vi "rad_RT Image Compare Dialog.vi"(5 "App Images Repository":path=path "c:/checksums.bin", 6 "Begin Automatically? (F)":bool, 7 "Temp Folder":path=path "C:/AppImages/_temp", 8 "error in (no error)":errorcluster, 9 "Operation":T4=enum."Compare Two Local Images", 10 "Target settings":T1={"Hostname"="", "Serial number"="", "Product name"="", "Product code"=0, "System status"="", "Credential type"=enum."None/Unlocked", "User added?"=FALSE, "Primary NIC"={"MAC address"="", "IP Address Request Mode"=2, "IP address"="", "Subnet mask"="", "Gateway"="", "DNS server"=""}} {"Primary NIC"."IP Address Request Mode" items=["Static"=1, "DHCP/Link-Local"=2, "Link-Local Only"=4, "DHCP Only"=8]}, 11 "Original Image Path":path) -> (0 "error out":errorcluster)   [LabVIEW 2020]
uses:
  TypeDefs/rad_Comparison Modes.ctl
  Targets/TypeDefs/rad_Target Information.ctl
  Targets/TypeDefs/rad_Target Network Settings.ctl
  Util/FP Control/FP Control Functions.ctl
  <vilib>/Utility/miscctls.llb/LVRowAndColumnUnsignedTypeDef.ctl
panel:
  in  "Compare Images":bool
  out "Results Table":i32(listbox)
  in  "Exit Notifier":bool
  in  "Ignore Automatically Updated Files":bool=TRUE
  in  "Comparison Image Path":path=path "c:/checksums.bin"
  in  "State Variables":T3
  in  "RT Target IP":string caption="RT Target - IP Address or Name"
  in  "Close":bool
  in  "Compare Files":bool
  # "Red software indicates different components"
  # "Blue software indicates different versions"
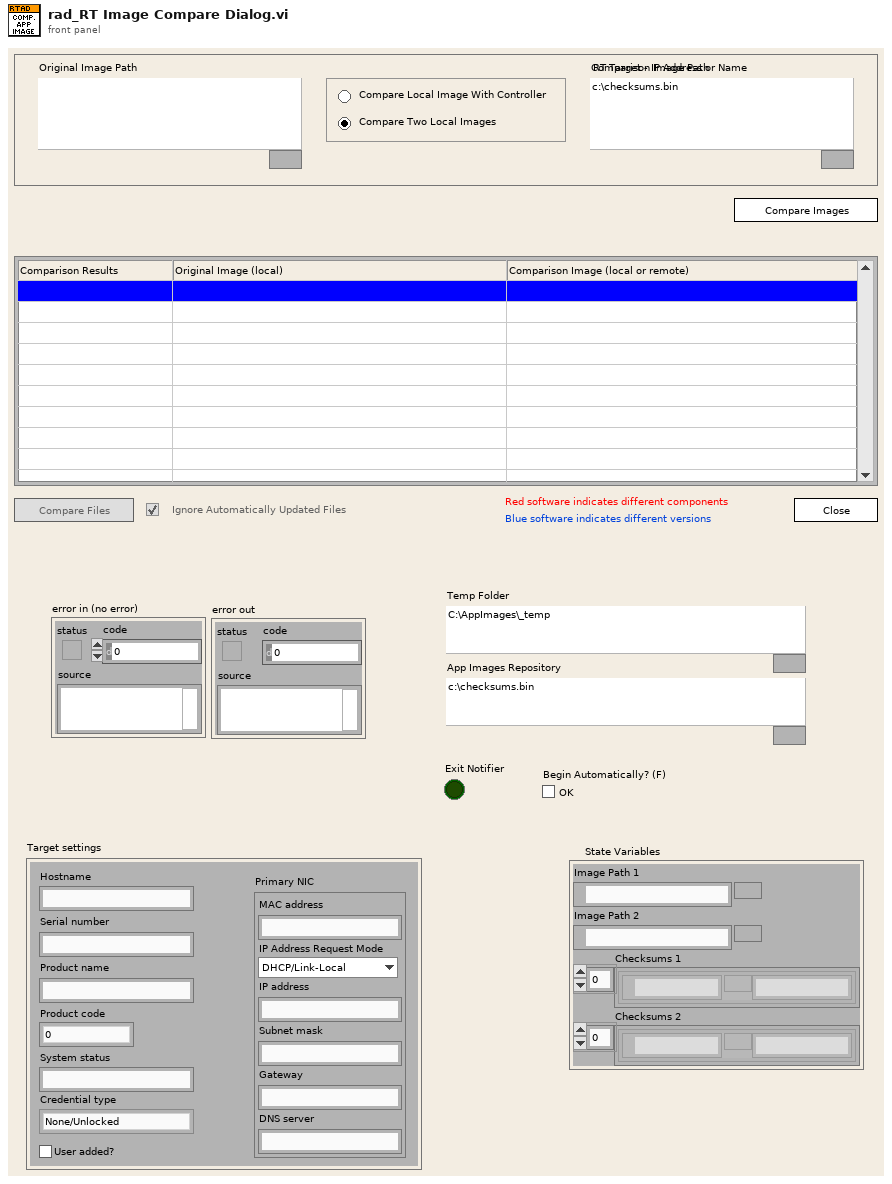
[diagram p1: front panel]
types:
  T1 = typedef "rad_Target Information.ctl" = cluster{"Hostname":string, "Serial number":string, "Product name":string, "Product code":i32, "System status":string, "Credential type":enum16{"None/Unlocked", "FTP Password", "NIAuth Credentials"}, "User added?":bool, "Primary NIC":T2}
  T2 = typedef "rad_Target Network Settings.ctl" = cluster{"MAC address":string, "IP Address Request Mode":i32, "IP address":string, "Subnet mask":string, "Gateway":string, "DNS server":string}
  T3 = cluster{"Image Path 1":path, "Image Path 2":path, "Checksums 1":cluster{path, string}[], "Checksums 2":cluster{path, string}[]}
  T4 = typedef "rad_Comparison Modes.ctl" = enum32{"Compare Local Image With Controller", "Compare Two Local Images"}
  T5 = typedef "LVRowAndColumnUnsignedTypeDef.ctl" = cluster{"Row":u32, "Column":u32}
  T6 = typedef "FP Control Functions.ctl" = enum16{"Open", "Close", "Bring To Front", "Center"}
  T7 = enum8{"Enabled", "Disabled", "Disabled and Grayed Out"}
  T8 = typedef "rad_Application Image Properties.ctl" = cluster{"Name":string, "Version":string, "Time":timestamp, "Description":string, "Key":string, "Chassis":string, "FPGA Properties":T9, "Model":string, "Retrieve":string[], "Deploy":string[], "Installed Software":string[]}
  T9 = typedef "rad_FPGA Properties.ctl" = T10[]
  T10 = typedef "rad_FPGA Flash Properties.ctl" = cluster{"Resource Name":string, "Path":path}
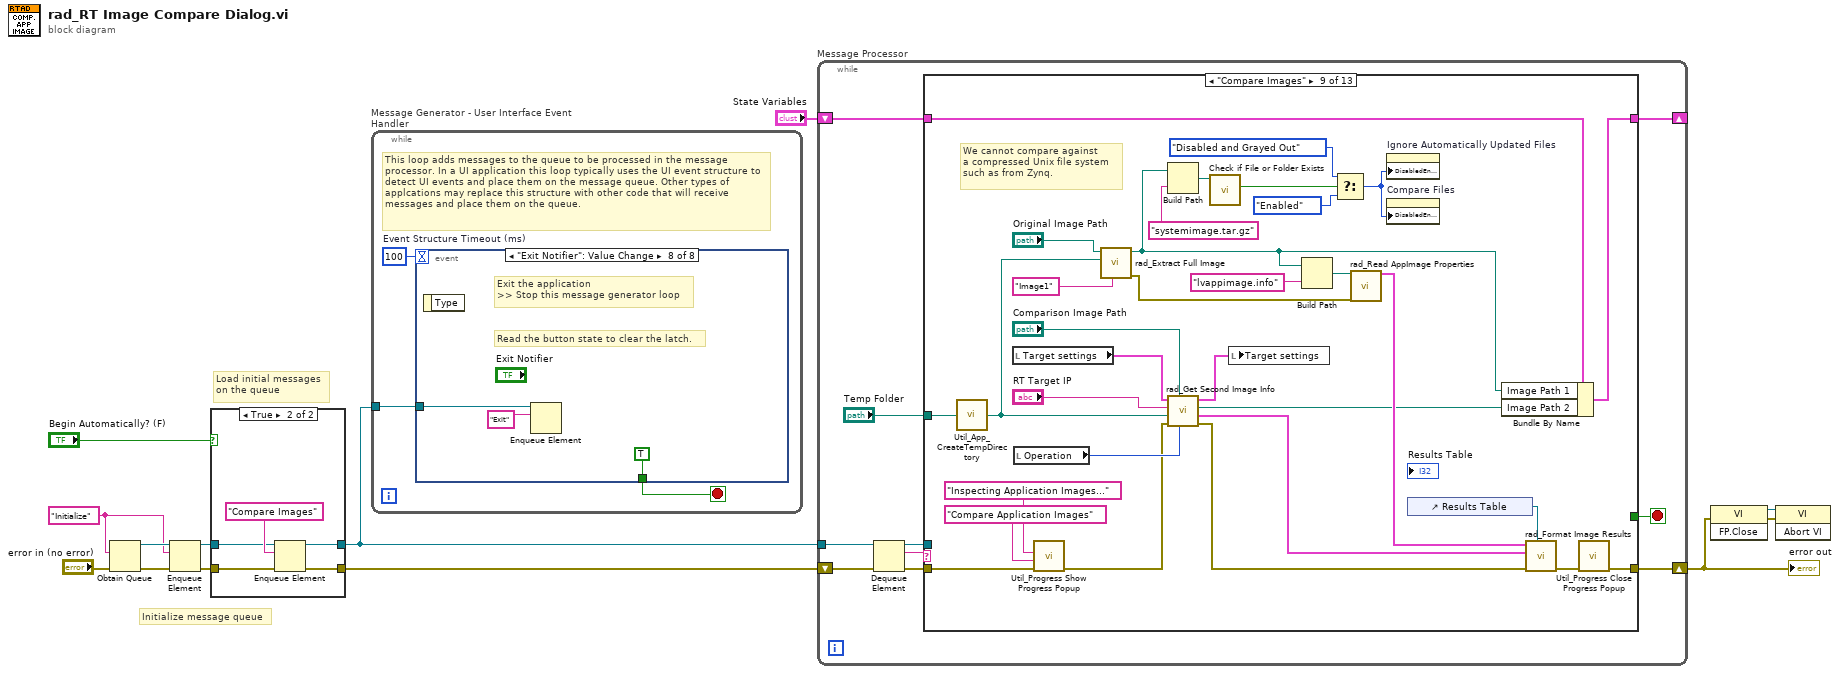
[diagram p0: block diagram]
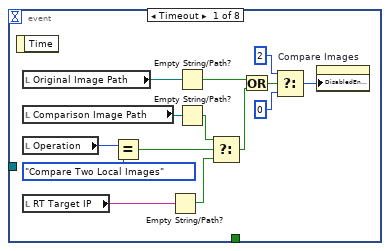
[diagram p3: hidden frame]
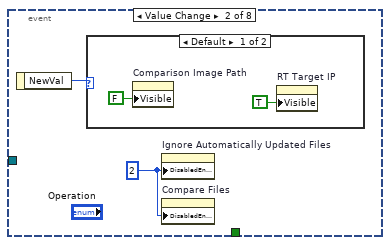
[diagram p4: hidden frame]
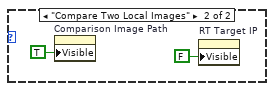
[diagram p5: hidden frame]
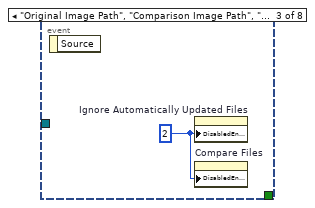
[diagram p6: hidden frame]
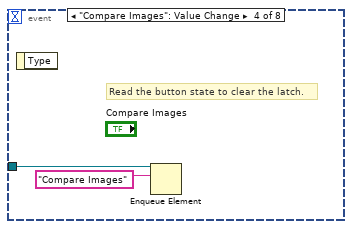
[diagram p7: hidden frame]
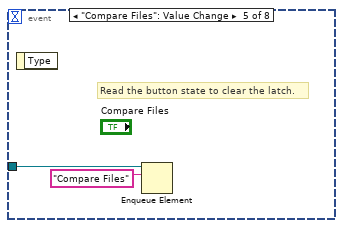
[diagram p8: hidden frame]
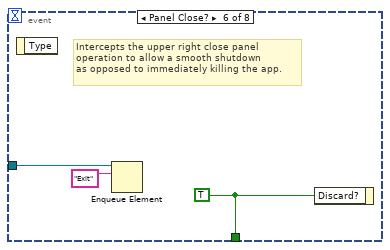
[diagram p9: hidden frame]
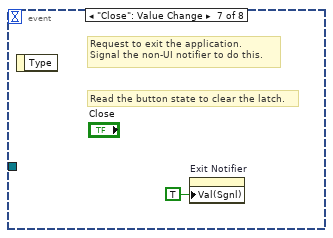
[diagram p10: hidden frame]
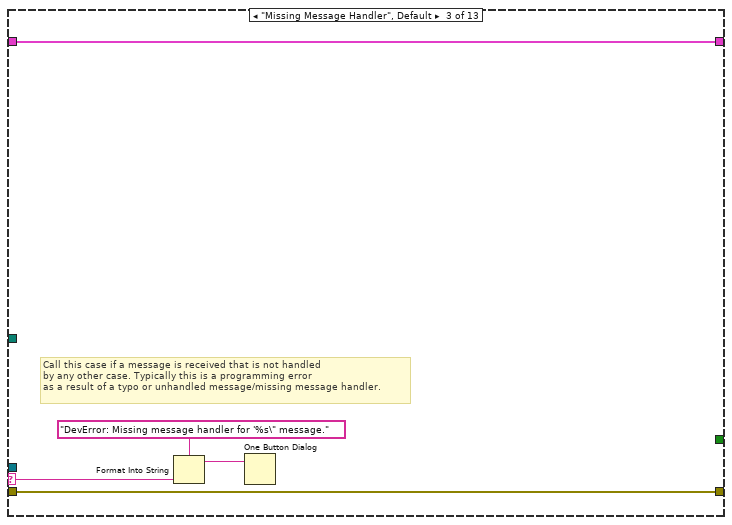
[diagram p13: hidden frame]
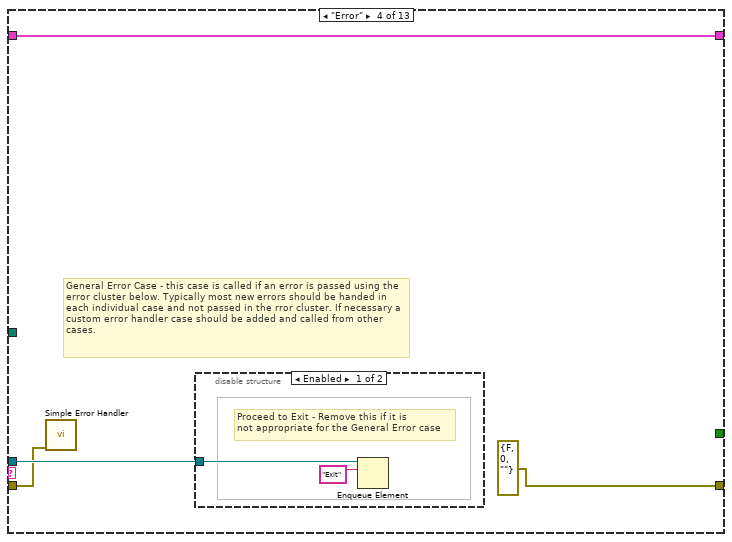
[diagram p14: hidden frame]
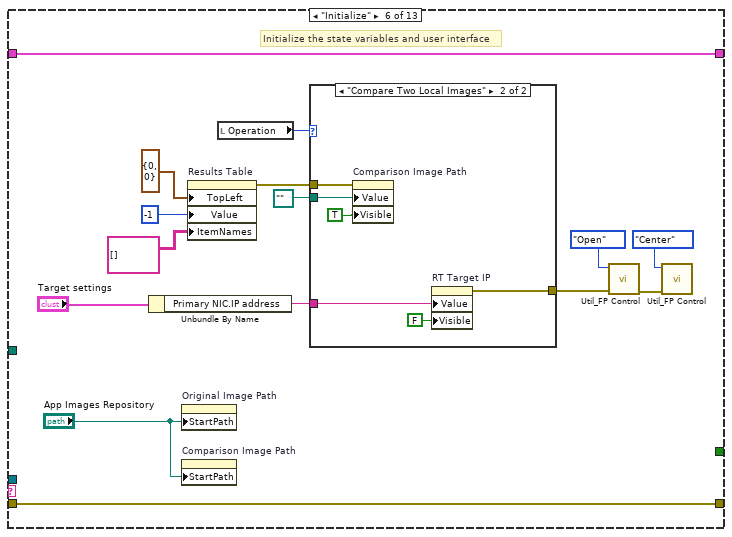
[diagram p17: hidden frame]
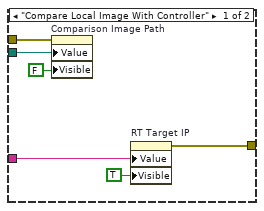
[diagram p18: hidden frame]
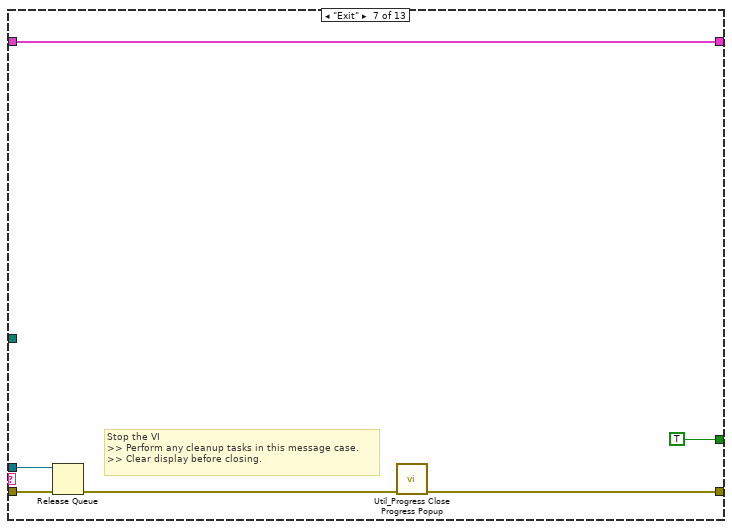
[diagram p19: hidden frame]
diagram:
  w5 = "Initialize"
  # "Initialize message queue"
  # "Load initial messages\non the queue"
  n1 = Obtain Queue(element data type=w5, error in (no error)="error in (no error)") -> (queue out=w7:refnum<queue>, error out=w6:errorcluster)  [unwired: 3 in, 1 out]
  n2 = Enqueue Element(queue=w7, element=w5, error in (no error)=w6) -> (queue out=w4:refnum<queue>, error out=w3:errorcluster)  [unwired: 1 in, 1 out]
  n3 = case shown="True" "Begin Automatically? (F)" {
    tunnel: w4 -> [w14 w19]
    tunnel: w3 -> [w15 w16]
    tunnel: [w15 w17] -> w2
    tunnel: [w14 w18] -> w1
    frame False {
    }
    frame True {
      n4 = Enqueue Element(queue=w19, element="Compare Images", error in (no error)=w16) -> (queue out=w18:refnum<queue>, error out=w17:errorcluster)  [unwired: 1 in, 1 out]
    }
  }
  n5 = while "Message Generator - User Interface Event Handler" {
    tunnel: w1 -> [w21]
    stop <- w22 stop-if-true
    w23 = 100  # Event Structure Timeout (ms)
    # "This loop adds messages to the queue to be processed in the message processor. In a UI application this loop typically uses the UI event structure to detect UI events and place them on the message queue. Other types of applcations may replace this structure with other code that will receive messages and place them on the queue."
    n6 = event shown="[7] \"Exit Notifier\": Value Change" {
      selector: _ -> [_ _ _ _ _ _ _ _]
      dyn-events: _ -> [_ _ _ _ _ _ _ _]
      timeout: w23 -> [_ _ _ _ _ _ _ _]
      tunnel: [_ _ _ _ _ w51 _ TRUE ("Discard?")] -> w22
      tunnel: w21 -> [_ _ _ w45 w48 w49 _ w53]
      event Timeout {
        n7 = event-data() -> ()  [unwired: 2 out]
        n8 = local read "Original Image Path"() -> (w27:path)
        n9 = local read "Comparison Image Path"() -> (w24:path)
        n10 = local read "Operation"() -> (w37:T4)
        n11 = local read "RT Target IP"() -> (w28:string)
        n12 = Equal?(x=w37, y=rad_Comparison_Modes."Compare Two Local Images") -> (x = y?=w35:bool)
        n13 = Empty String/Path?(string/path=w28) -> (empty?=w29:bool)
        n14 = Empty String/Path?(string/path=w27) -> (empty?=w26:bool)
        n15 = Empty String/Path?(string/path=w24) -> (empty?=w25:bool)
        n16 = Select(t=w25, s=w35, f=w29) -> (s? t:f=w34:bool)
        n17 = Or(x=w26, y=w34) -> (x .or. y?=w33:bool)
        n18 = Select(t=2, s=w33, f=0) -> (s? t:f=w30:i32)
        n19 = property on="Compare Images" class="Bool"("DisabledEnum"=w30) -> ()  [unwired: 2 in, 2 out]
      }
      event Value Change {
        w38 = 2
        n20 = event-data() -> ("NewVal"=w39:T4)  [unwired: 1 out]
        n21 = case shown="Default" w39 {
          frame Default {
            n22 = property on="Comparison Image Path" class="Path"("Visible"=FALSE) -> ()  [unwired: 2 in, 2 out]
            n23 = property on="RT Target IP" class="Str"("Visible"=TRUE) -> ()  [unwired: 2 in, 2 out]
          }
          frame "Compare Two Local Images" {
            n24 = property on="Comparison Image Path" class="Path"("Visible"=TRUE) -> ()  [unwired: 2 in, 2 out]
            n25 = property on="RT Target IP" class="Str"("Visible"=FALSE) -> ()  [unwired: 2 in, 2 out]
          }
        }
        n26 = property on="Ignore Automatically Updated Files" class="Bool (strict)"("DisabledEnum"=w38) -> ()  [unwired: 2 in, 2 out]
        n27 = property on="Compare Files" class="Bool"("DisabledEnum"=w38) -> ()  [unwired: 2 in, 2 out]
      }
      event "Original Image Path", "Comparison Image Path", "RT Target IP": Value Change {
        w44 = 2
        n28 = event-data() -> ()  [unwired: 2 out]
        n29 = property on="Ignore Automatically Updated Files" class="Bool (strict)"("DisabledEnum"=w44) -> ()  [unwired: 2 in, 2 out]
        n30 = property on="Compare Files" class="Bool"("DisabledEnum"=w44) -> ()  [unwired: 2 in, 2 out]
      }
      event "Compare Images": Value Change {
        # "Read the button state to clear the latch."
        n31 = event-data() -> ()  [unwired: 2 out]
        n32 = Enqueue Element(queue=w45, element="Compare Images") -> ()  [unwired: 2 in, 3 out]
      }
      event "Compare Files": Value Change {
        # "Read the button state to clear the latch."
        n33 = event-data() -> ()  [unwired: 2 out]
        n34 = Enqueue Element(queue=w48, element="Compare Files") -> ()  [unwired: 2 in, 3 out]
      }
      event Panel Close? {
        w51 = TRUE ("Discard?")
        # "Intercepts the upper right close panel\noperation to allow a smooth shutdown\nas opposed to immediately killing the app."
        n35 = event-data() -> ()  [unwired: 2 out]
        n36 = Enqueue Element(queue=w49, element="Exit") -> ()  [unwired: 2 in, 3 out]
        n37 = event-data("Discard?"=w51) -> ()  [unwired: 1 in, 1 out]
      }
      event "Close": Value Change {
        # "Read the button state to clear the latch."
        # "Request to exit the application.\nSignal the non-UI notifier to do this."
        n38 = event-data() -> ()  [unwired: 2 out]
        n39 = property on="Exit Notifier" class="Bool (strict)"("Val(Sgnl)"=TRUE ("Value (Signaling)")) -> ()  [unwired: 2 in, 2 out]
      }
      event "Exit Notifier": Value Change {
        # "Read the button state to clear the latch."
        # "Exit the application\n>> Stop this message generator loop"
        n40 = event-data() -> ()  [unwired: 2 out]
        n41 = Enqueue Element(queue=w53, element="Exit") -> ()  [unwired: 2 in, 3 out]
      }
    }
  }
  n42 = while "Message Processor" {
    shift-left: w2 -> [w60]
    shift-right: [w63] -> w8
    tunnel: w1 -> [w61]
    shift-left: "State Variables" -> [w65]
    shift-right: [w64] -> _
    stop <- w56 stop-if-true
    n43 = Dequeue Element(queue=w61, error in (no error)=w60) -> (queue out=w62:refnum<queue>, element=w58:string, error out=w59:errorcluster)  [unwired: 1 in, 1 out]
    n44 = case shown="\"Compare Images\"" w58 {
      selector: w58 -> [_ _ w72 _ _ _ _ _ _ _ _ _ _]
      tunnel: [w67 w69 w74 w78 w82 w97 w115 w117 w148 w150 w192 w208 w216] -> w64
      tunnel: w65 -> [w67 w69 w74 w78 w82 w97 w115 w117 w149 w150 w193 w208 w216]
      tunnel: w62 -> [_ _ _ w76 _ _ w113 _ _ w153 w191 w207 _]
      tunnel: w59 -> [w66 w68 w73 w75 w81 w96 w114 w116 w125 w156 w181 w194 w217]
      tunnel: [w66 w68 w73 errorcluster {"status"=FALSE, "code"=0, "source"=""} ("error out") w81 w96 w111 w116 w126 w155 w183 w199 w213] -> w63
      tunnel: "Temp Folder" -> [_ _ _ _ _ _ _ _ w145 _ _ _ w219]
      tunnel: [_ _ _ _ _ _ TRUE _ _ _ _ _ _] -> w56
      frame "---------- Framework Operations ----------" {
        # "Dummy case to add a seperator in the Case Structure menu"
      }
      frame "", "Idle" {
        # "Idle Case - this case is called after a Timeout on the Get Next Message from Queue VI, if no new messages are present on the queue. This case can be used for housekeeping tasks such as updating the UI."
      }
      frame "Missing Message Handler", Default {
        # "Call this case if a message is received that is not handled \nby any other case. Typically this is a programming error\nas a result of a typo or unhandled message/missing message handler."
        n45 = Format Into String(format string="DevError: Missing message handler for '%s\" message." ("message"), w72) -> (resulting string=w70:string)  [unwired: 2 in, 1 out]
        n46 = One Button Dialog(message=w70) -> ()  [unwired: 2 out]
      }
      frame "Error" {
        # "General Error Case - this case is called if an error is passed using the error cluster below. Typically most new errors should be handed in each individual case and not passed in the rror cluster. If necessary a custom error handler case should be added and called from other cases."
        n47 = call <vilib>:"Simple Error Handler.vi"("error in (no error)"=w75) -> ()  [unwired: 1 in, 8 out]
        n48 = disable-structure shown="Enabled" {
          disable-tunnel: w76 -> [w80 _]
          frame Enabled {
            # "Proceed to Exit - Remove this if it is\nnot appropriate for the General Error case"
            n49 = Enqueue Element(queue=w80, element="Exit") -> ()  [unwired: 2 in, 3 out]
          }
          frame Disabled {
          }
        }
      }
      frame "---------- Generic Operations ----------" {
        # "Dummy case to add a seperator in the Case Structure menu"
      }
      frame "Initialize" {
        # "Initialize the state variables and user interface"
        n50 = Unbundle By Name("Target settings") -> ("Primary NIC.IP address"=w87:string)
        n51 = property on="Original Image Path" class="Path"("StartPath"="App Images Repository") -> ()  [unwired: 2 in, 2 out]
        n52 = property on="Comparison Image Path" class="Path"("StartPath"="App Images Repository") -> ()  [unwired: 2 in, 2 out]
        n53 = property on="Results Table" class="MCListbox (strict)"("TopLeft"=T5 {"Row"=0, "Column"=0} ("Top Left Visible Cell"), "Value"=-1 ("Results Table"), "ItemNames"=string[][] [] ("Item Names")) -> (error out=w83:errorcluster)  [unwired: 2 in, 1 out]
        n54 = local read "Operation"() -> (w88:T4)
        n55 = case shown="\"Compare Two Local Images\"" w88 {
          tunnel: [w103 w109] -> w93
          tunnel: path "" ("Value (Signaling)") -> [w100 w106]
          tunnel: w87 -> [w99 w105]
          tunnel: w83 -> [w98 w104]
          frame "Compare Local Image With Controller" {
            n56 = property on="Comparison Image Path" class="Path"(error in=w98, "Value"=w100, "Visible"=FALSE) -> ()  [unwired: 1 in, 2 out]
            n57 = property on="RT Target IP" class="Str"("Value"=w99, "Visible"=TRUE) -> (error out=w103:errorcluster)  [unwired: 2 in, 1 out]
          }
          frame "Compare Two Local Images" {
            n58 = property on="Comparison Image Path" class="Path"(error in=w104, "Value"=w106, "Visible"=TRUE) -> ()  [unwired: 1 in, 2 out]
            n59 = property on="RT Target IP" class="Str"("Value"=w105, "Visible"=FALSE) -> (error out=w109:errorcluster)  [unwired: 2 in, 1 out]
          }
        }
        n60 = call "Util_FP Control.vi"("error in (no error)"=w93, "Function"=FP_Control_Functions."Open") -> ("error out"=w91:errorcluster)  [unwired: 9 out]
        n61 = call "Util_FP Control.vi"("error in (no error)"=w91, "Function"=FP_Control_Functions."Center") -> ()  [unwired: 10 out]
      }
      frame "Exit" {
        # "Stop the VI\n>> Perform any cleanup tasks in this message case.\n>> Clear display before closing."
        n62 = Release Queue(queue=w113, error in (no error)=w114) -> (error out=w112:errorcluster)  [unwired: 1 in, 2 out]
        n63 = call "Util_Progress Close Progress Popup.vi"("error in (no error)"=w112) -> ("error out"=w111:errorcluster)  [unwired: 10 in]
      }
      frame "---------- Application Operations ----------" {
        # "Dummy case to add a seperator in the Case Structure menu"
      }
      frame "Compare Images" {
        # "We cannot compare against\na compressed Unix file system\nsuch as from Zynq."
        n64 = call "Util_App_CreateTempDirectory.vi"("TempFolderPath"=w145) -> ("TempFolderPath_out"=w135:path)
        n65 = local read "Target settings"() -> (w122:T1)
        n66 = local read "Operation"() -> (w144:T4)
        n67 = call "Util_Progress Show Progress Popup.vi"("error in (no error)"=w125, "Title"="Compare Application Images", "Message"="Inspecting Application Images...") -> ("error out"=w124:errorcluster)  [unwired: 8 in]
        n68 = call "rad_Extract Full Image.vi"("Subfolder (lvappimage.contents)"="Image1" ("name or relative path"), "App Image Temp Folder"=w135, "Zipped App Image File Path"="Original Image Path") -> ("error out"=w123:errorcluster, "Unzipped App Image Folder Path"=w128:path)  [unwired: 7 in]
        n69 = Build Path(base path=w128, name or relative path="systemimage.tar.gz") -> (appended path=w131:path)
        n70 = call "rad_Get Second Image Info.vi"("Operation"=w144, "Comparison Image Path"="Comparison Image Path", "error in (no error)"=w124, "TempFolder Path"=w135, "RT Target IP"="RT Target IP", "Target settings in"=w122) -> ("error out"=w141:errorcluster, "AppImage Properties"=w120:T8, "Unzipped App Image Folder Path"=w119:path, "Target settings out"=w118:T1)  [unwired: 2 in]
        n71 = call <vilib>:"Check if File or Folder Exists.vi"("path"=w131) -> ("file or folder exists?"=w130:bool)  [unwired: 8 in, 2 out]
        n72 = local write "Target settings"(w118) -> ()
        n73 = Build Path(base path=w128, name or relative path="lvappimage.info") -> (appended path=w138:path)
        n74 = Select(t=T7."Disabled and Grayed Out" ("Disabled"), s=w130, f=T7."Enabled" ("Disabled")) -> (s? t:f=w134:T7)
        n75 = call "rad_Read AppImage Properties.vi"("AppImage Properties Path"=w138, "error in (no error)"=w123) -> ("AppImage Properties"=w137:T8)  [unwired: 12 in, 5 out]
        n76 = property on="Ignore Automatically Updated Files" class="Bool (strict)"("DisabledEnum"=w134) -> ()  [unwired: 2 in, 2 out]
        n77 = property on="Compare Files" class="Bool"("DisabledEnum"=w134) -> ()  [unwired: 2 in, 2 out]
        n78 = control-ref of="Results Table"() -> (w140:refnum<vi>)
        n79 = Bundle By Name(cluster=w149, "Image Path 1"=w128, "Image Path 2"=w119) -> (w148:T3)
        n80 = call "rad_Format Image Results.vi"("Results listbox"=w140, "error in (no error)"=w141, "AppImage 2"=w120, "AppImage 1"=w137) -> ("error out"=w127:errorcluster)  [unwired: 7 in]
        n81 = call "Util_Progress Close Progress Popup.vi"("error in (no error)"=w127) -> ("error out"=w126:errorcluster)  [unwired: 10 in]
      }
      frame "Compare Files" {
        n82 = local read "Operation"() -> (w151:T4)
        n83 = call "Util_Progress Show Progress Popup.vi"("error in (no error)"=w156, "Title"="Compare Application Images", "Message"="Inspecting File Systems...") -> ()  [unwired: 8 in, 1 out]
        n84 = case shown="\"Compare Local Image With Controller\"" w151 {
          tunnel: [w176 w178] -> w154
          tunnel: w156 -> [w177 w178]
          tunnel: [w175 _] -> w152
          tunnel: w150 -> [w174 _]
          frame "Compare Local Image With Controller" {
            # "The original image was already\nexpanded, but we still need to\nget the target's image."
            n85 = Unbundle By Name(w174) -> ("Image Path 2"=w173:path)
            n86 = local read "Target settings"() -> (w172:T1)
            n87 = call "rad_Retrieve Image Wrapper.vi"("error in (no error)"=w177, "image file path"=w173, "Target settings"=w172) -> ("error out"=w176:errorcluster, "Canceled"=w175:bool)  [unwired: 7 in]
          }
          frame "Compare Two Local Images" {
            # "Both file systems were\nalready expanded during the\nCompare Images step."
          }
        }
        n88 = case shown="No Error" w154 {
          selector: w154 -> [w161 w171]
          tunnel: [w162 w171] -> w155
          tunnel: w153 -> [w160 _]
          tunnel: w152 -> [w159 _]
          frame No Error {
            n89 = case shown="False" w159 {
              tunnel: [w165 w169] -> w162
              tunnel: w161 -> [w164 w170]
              tunnel: w160 -> [w163 w167]
              frame False {
                n90 = Enqueue Element(queue=w163, element="Create Checksums", error in (no error)=w164) -> (error out=w165:errorcluster)  [unwired: 1 in, 2 out]
              }
              frame True {
                n91 = Enqueue Element(queue=w167, element="Cleanup", error in (no error)=w170) -> (error out=w169:errorcluster)  [unwired: 1 in, 2 out]
              }
            }
          }
          frame Error {
          }
        }
      }
      frame "Create Checksums" {
        n92 = Unbundle By Name(w193) -> ("Image Path 1"=w179:path, "Image Path 2"=w180:path)
        n93 = call "rad_Calculate Checksum.vi"("error in"=w181, "Ignore tmp Files"="Ignore Automatically Updated Files", "Image Base Folder"=w179) -> ("error out"=w185:errorcluster, "Checksums"=w189:cluster{path, "MD5 message-digest":string}[])  [unwired: 6 in, 1 out]
        n94 = call "rad_Calculate Checksum.vi"("error in"=w181, "Ignore tmp Files"="Ignore Automatically Updated Files", "Image Base Folder"=w180) -> ("error out"=w186:errorcluster, "Checksums"=w188:cluster{path, "MD5 message-digest":string}[])  [unwired: 6 in, 1 out]
        n95 = Enqueue Element(queue=w191, element="Compare" ("Message Name"), error in (no error)=w181) -> (error out=w187:errorcluster)  [unwired: 1 in, 2 out]
        n96 = Bundle By Name(cluster=w193, "Checksums 1"=w189, "Checksums 2"=w188) -> (w192:T3)
        n97 = Merge Errors(w185, w186, w187) -> (w182:errorcluster)
        n98 = call "Util_Progress Close Progress Popup.vi"("error in (no error)"=w182) -> ("error out"=w183:errorcluster)  [unwired: 10 in]
      }
      frame "Compare" {
        n99 = call "Util_Progress Show Progress Popup.vi"("error in (no error)"=w194, "Title"="Compare Application Images", "Message"="Comparing Application Checksums...") -> ("error out"=w195:errorcluster)  [unwired: 8 in]
        n100 = Unbundle By Name(w208) -> ("Checksums 1"=w204:cluster{path, string}[], "Checksums 2"=w205:cluster{path, string}[])
        n101 = Enqueue Element(queue=w207, element="Cleanup" ("Message Name"), error in (no error)=w195) -> (error out=w199:errorcluster)  [unwired: 1 in, 2 out]
        n102 = call "rad_Compare Checksums.vi"("Checksums 2"=w205, "Checksums 1"=w204) -> ("Files In 2 Only"=w200:path[], "Files In 1 Only"=w201:path[], "Modified Files"=w202:path[], "Identical?"=w203:bool)  [unwired: 6 out]
        n103 = call "Util_Progress Close Progress Popup.vi"("error in (no error)"=w199) -> ("error out"=w198:errorcluster)  [unwired: 10 in]
        n104 = case shown="False" w203 {
          tunnel: w202 -> [w211 _]
          tunnel: w201 -> [w210 _]
          tunnel: w200 -> [w209 _]
          tunnel: w198 -> [_ _]
          frame False {
            n105 = call "rad_View Comparison Results.vi"("Files Found Only In New Image"=w209, "Files Found Only In Original Image"=w210, "Modified Files"=w211) -> ()  [unwired: 8 in, 1 out]
          }
          frame True {
            n106 = One Button Dialog(message="RT Image Verified Successfully.\nThe Two Images Are Identical.") -> ()  [unwired: 1 in, 1 out]
          }
        }
      }
      frame "Cleanup" {
        n107 = Delete(path (use dialog)=w219, entire hierarchy (F)=TRUE, error in=w217) -> (error out=w214:errorcluster)  [unwired: 2 in, 2 out]
        n108 = local read "Begin Automatically? (F)"() -> (w215:bool)
        n109 = case shown="True" w215 {
          frame False {
          }
          frame True {
            n110 = property on="Exit Notifier" class="Bool (strict)"("Val(Sgnl)"=TRUE ("Value (Signaling)")) -> ()  [unwired: 2 in, 2 out]
          }
        }
        n111 = call <vilib>:"Clear Errors.vi"("error in (no error)"=w214) -> ("error out"=w213:errorcluster)  [unwired: 5 in, 1 out]
      }
    }
  }
  "error out" <- w8
  n112 = invoke class="VI" method="FP.Close"(error in=w8) -> (reference out=w10:refnum<vi>, error out=w9:errorcluster)  [unwired: 2 in, 1 out]
  n113 = invoke class="VI" method="Abort VI"(reference=w10, error in=w9) -> ()  [unwired: 1 in, 3 out]
